vi "Asylum_ReadScanSizeAndOffset_fromLUT.vi"(11 "Notes LUT":variant) -> (0 "Y Offset":dbl, 1 "X Offset":dbl, 2 "Y Range":dbl, 3 "X Range":dbl)   [LabVIEW 2019]
panel:
  out "error out":errorcluster
  in  "error in":errorcluster
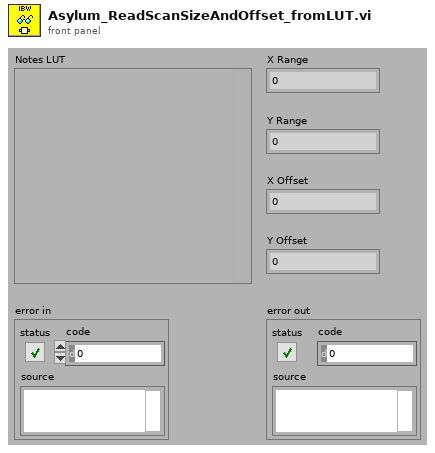
[diagram p1: front panel]
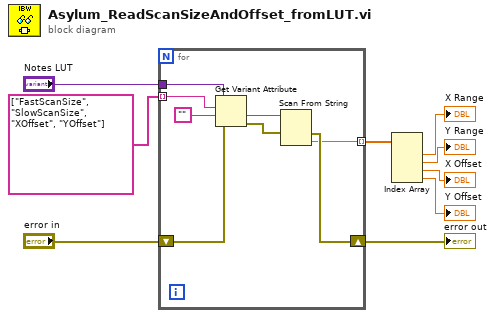
[diagram p0: block diagram]
diagram:
  n1 = for {
    tunnel: string[] ["FastScanSize", "SlowScanSize", "XOffset", "YOffset"] -> [w14] mode=indexing
    tunnel: "Notes LUT" -> [w10]
    tunnel: [w12] -> w6 mode=indexing
    shift-right: [w16] -> w8
    shift-left: "error in" -> [w17]
    n2 = Get Variant Attribute(Variant=w10, name=w14, default value (empty Variant)="", error in=w17) -> (value=w11:string, error out=w15:errorcluster)  [unwired: 2 out]
    n3 = Scan From String(input string=w11, error in=w15) -> (error out=w16:errorcluster, output 1=w12:dbl)  [unwired: 3 in, 2 out]
  }
  "error out" <- w8
  n4 = Index Array(array=w6) -> (element #1=→"X Range":dbl, element #2=→"Y Range":dbl, element #3=→"X Offset":dbl, element #4=→"Y Offset":dbl)  [unwired: 4 in]
